vi "rs3 showError.vi"(8 "error in (no error)":errorcluster, 11 "error":u64) -> (0 "error out":errorcluster, 1 "error message":string, 2 "Failed args":string, 3 "Failed Function":string, 5 "Error summary":string)   [LabVIEW 2018, in "libRealSense3.lvlib"]
doc: "Describes the Error received from any any previous libRealSense VI"
uses:
  libRealSense3.lvlib
panel:
  # "RS3 Show Errors"
  # "(C) Intel Corp.,  AGJ"
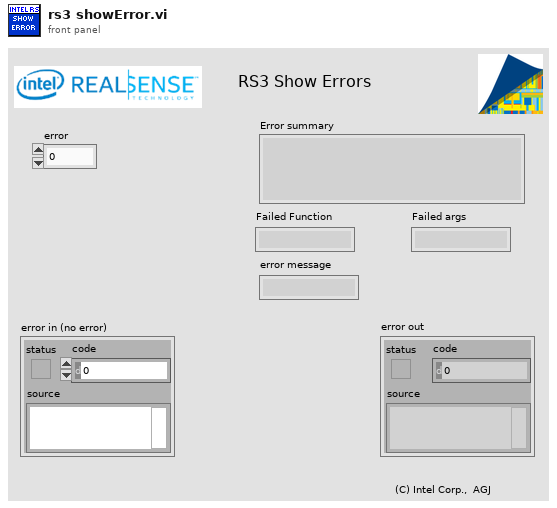
[diagram p1: front panel]
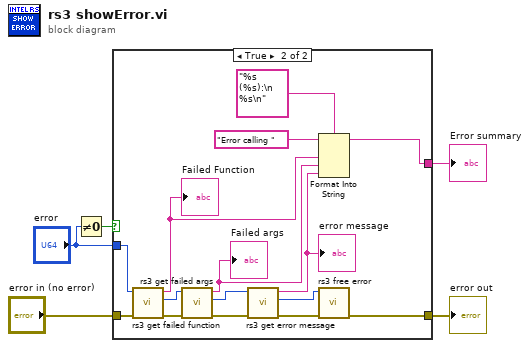
[diagram p0: block diagram]
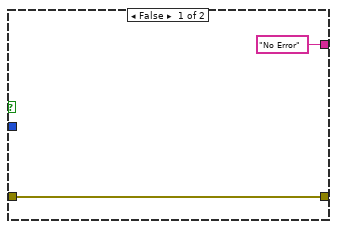
[diagram p2: hidden frame]
diagram:
  n1 = Not Equal To 0?(x="error") -> (x != 0?=w2:bool)
  n2 = case shown="True" w2 {
    tunnel: "error in (no error)" -> [w7 w22]
    tunnel: [w7 w21] -> w4
    tunnel: "error" -> [_ w19]
    tunnel: ["No Error" w18] -> w3
    frame False {
    }
    frame True {
      n3 = call "rs3 get failed function.vi"("error in (no error)"=w22, "error in"=w19) -> (0:"error out"=w8:errorcluster, 2:"error out"=w11:u64, "Failed Function"=w15:string)  [unwired: 7 in]
      "Failed Function" <- w15
      n4 = call "rs3 get failed args.vi"("error in (no error)"=w8, "error in"=w11) -> (0:"error out"=w9:errorcluster, 2:"error out"=w12:u64, "Failed args"=w16:string)  [unwired: 7 in]
      "Failed args" <- w16
      n5 = call "rs3 get error message.vi"("error in (no error)"=w9, "error in"=w12) -> (0:"error out"=w10:errorcluster, 2:"error out"=w20:u64, "error message"=w17:string)  [unwired: 7 in]
      "error message" <- w17
      n6 = Format Into String(format string="%s (%s):\n %s\n", initial string="Error calling ", w15, w16, w17) -> (resulting string=w18:string)  [unwired: 1 in, 1 out]
      n7 = call "rs3 free error.vi"("error in (no error)"=w10, "error in"=w20) -> ("error out 2"=w21:errorcluster)  [unwired: 8 in, 1 out]
    }
  }
  "Error summary" <- w3
  "error out" <- w4
